vi "DefaultFromIni.vi"(8 "error in (no error)":errorcluster, 11 "C37.118 Sim in":refnum<class "C37.118 Sim.lvclass">) -> (0 "error out":errorcluster, 3 "C37.118 Sim out":refnum<class "C37.118 Sim.lvclass">)   [LabVIEW 2018, in "SensorPlugins.lvlib" / "C37.118 Sim.lvclass"]
uses:
  C37.118 Sim.lvclass
  C:/Program Files (x86)/National Instruments/LabVIEW 2018/user.lib/NIST/BaseClasses/BasePlugin_class/BasePlugin.lvclass
  <userlib>/NIST/BaseClasses/BasePlugin_class/BasePlugin.lvclass/BasePlugin.ctl
  FGen/MemberClasses/FunctionBaseClass/FunctionBase.lvclass
  C37.118 Sim.lvclass/C37.118 Sim.ctl
  <userlib>/NIST/BaseClasses/BasePlugin_class/Accessors/Read PluginIniFilePath.vi
  Accessors/Write FunctionIniFilePath.vi
  Accessors/Write Time.vi
  Accessors/Write Function.vi
  <vilib>/Utility/error.llb/Error Cluster From Error Code.vi
  PmuBaseClass/PmuBase.lvclass
  <vilib>/ErrorRing/Error Ring.xnode
  <vilib>/Utility/config.llb/NI_LVConfig.lvlib
  <userlib>/NIST/BaseClasses/Object_class/BaseObject.lvclass
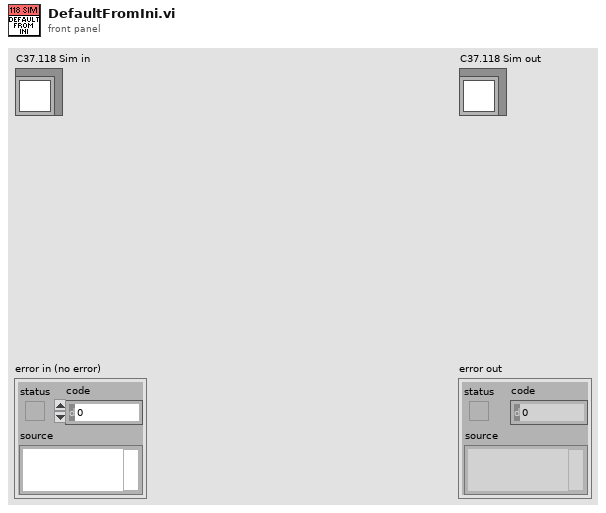
[diagram p1: front panel]
types:
  T1 = typedef "NI_LVConfig.lvlib/Config Data RefNum.ctl" = refnum<k1>
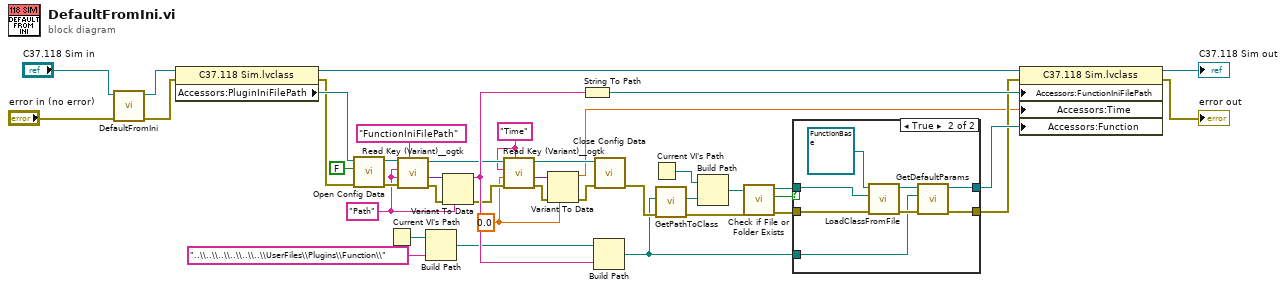
[diagram p0: block diagram]
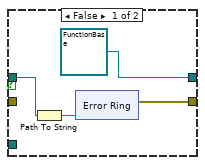
[diagram p2: hidden frame]
diagram:
  w6 = 0.0
  w8 = "Time" ("section")
  w13 = "Path" ("key (optional)")
  n1 = call-parent "DefaultFromIni.vi"("error in (no error)"="error in (no error)", "PmuBase in"="C37.118 Sim in") -> ("error out"=w37:errorcluster, "PmuBase out"=w41:refnum<class "C37.118 Sim.lvclass">)  [unwired: 8 in]
  n2 = property class="C37.118 Sim.lvclass"(reference=w41, error in=w37) -> (reference out=w38:refnum<class "C37.118 Sim.lvclass">, error out=w35:errorcluster, "Accessors:PluginIniFilePath"=w36:path)
  n3 = call <vilib>:"Open Config Data.vi"("error in (no error)"=w35, "create file if necessary (T)"=FALSE, "configuration file path"=w36) -> ("error out"=w33:errorcluster, "refnum"=w15:T1)  [unwired: 6 in, 1 out]
  n4 = Current VI's Path() -> (path=w12:path)
  n5 = call <userlib>:"Read Key (Variant)__ogtk.vi"("section"="FunctionIniFilePath", "error in (no error)"=w33, "type"=w13, "key (optional)"=w13, "refnum"=w15) -> ("error out"=w32:errorcluster, "key-value"=w30:variant, "refnum out"=w9:T1)  [unwired: 3 in, 1 out]
  n6 = Build Path(base path=w12, name or relative path="..\\..\\..\\..\\..\\..\\UserFiles\\Plugins\\Function\\") -> (appended path=w10:path)
  n7 = Variant To Data(error in=w32, type=w13, Variant=w30) -> (data=w20:string, error out=w7:errorcluster)
  n8 = call <userlib>:"Read Key (Variant)__ogtk.vi"("section"=w8, "error in (no error)"=w7, "type"=w6, "key (optional)"=w8, "refnum"=w9) -> ("error out"=w4:errorcluster, "key-value"=w3:variant, "refnum out"=w2:T1)  [unwired: 3 in, 1 out]
  n9 = Variant To Data(error in=w4, type=w6, Variant=w3) -> (data=w1:dbl, error out=w5:errorcluster)
  n10 = String To Path(string=w20) -> (path=w28:path)
  n11 = Build Path(base path=w10, name or relative path=w20) -> (appended path=w19:path)
  n12 = call <vilib>:"Close Config Data.vi"("error in (no error)"=w5, "refnum"=w2) -> ("error out"=w29:errorcluster)  [unwired: 8 in, 1 out]
  n13 = Current VI's Path() -> (path=w27:path)
  n14 = call <userlib>:"GetPathToClass.vi"("error in (no error)"=w29, "configuration file path"=w19) -> ("error IO"=w24:errorcluster, "PathToClass"=w26:path)  [unwired: 8 in]
  n15 = Build Path(base path=w27, name or relative path=w26) -> (appended path=w25:path)
  n16 = call <vilib>:"Check if File or Folder Exists.vi"("error in (no error)"=w24, "path"=w25) -> ("error out"=w23:errorcluster, "file or folder exists?"=w21:bool, "dup path"=w22:path)  [unwired: 7 in]
  n17 = case shown="True" w21 {
    tunnel: [w44 w55] -> w17
    tunnel: w23 -> [_ w60]
    tunnel: w22 -> [w43 w59]
    tunnel: w19 -> [_ w53]
    tunnel: [refnum<class "FunctionBase.lvclass"> refnum ("Functions.lvlib:FunctionBase.lvclass") w54] -> w18
    frame False {
      n18 = Path To String(path=w43) -> (string=w45:string)
      n19 = xnode "Error Ring"("parameter 0"=w45) -> ("error out"=w44:errorcluster)
    }
    frame True {
      n20 = call-dynamic "LoadClassFromFile.vi"("error in (no error)"=w60, "class path"=w59, "reference in"=refnum<class "FunctionBase.lvclass"> refnum ("Functions.lvlib:FunctionBase.lvclass")) -> ("error out"=w57:errorcluster, "reference out"=w56:refnum<class "FunctionBase.lvclass">)  [unwired: 7 in]
      n21 = call-dynamic "GetDefaultParams.vi"("error in (no error)"=w57, "Path"=w53, "FunctionBase in"=w56) -> ("error out"=w55:errorcluster, "FunctionBase out"=w54:refnum<class "FunctionBase.lvclass">)  [unwired: 7 in]
    }
  }
  n22 = property class="C37.118 Sim.lvclass"(reference=w38, error in=w17, "Accessors:FunctionIniFilePath"=w28, "Accessors:Time"=w1, "Accessors:Function"=w18) -> (reference out=→"C37.118 Sim out":refnum<class "C37.118 Sim.lvclass">, error out=→"error out":errorcluster)
